vi "RS485_Sensor_Data.vi"() -> ()   [LabVIEW 2016]
uses:
  <vilib>/Instr/_visa.llb/VISA Set IO Buffer Mask.ctl
  <vilib>/Instr/_visa.llb/VISA Flush IO Buffer Mask.ctl
  <vilib>/Analysis/NI_AALBase.lvlib
  GEN_2.lvlib
  <vilib>/Instr/_visa.llb/VISA Configure Serial Port (Instr).vi
  <vilib>/Analysis/1siggen.llb/Ramp Pattern by Delta.vi
  Sensor_GEN2_Config_Addr.ctl
  Sensor_GEN2_Stat_Addr.ctl
panel:
  in  "Limits 2":cluster{"F0":sgl, "F1":sgl}={"F0"=-0.5925, "F1"=-0.5925}
  in  "Write_Scales":bool
  in  "Write_offsets":bool
  in  "Limits":cluster{"F0":sgl, "F1":sgl}={"F0"=-62.0, "F1"=-401.0}
  in  "Write Configs":bool
  out "Theta_dot":cluster{"Mean":dbl, "Std":dbl}={"Mean"=nan, "Std"=-0.0} {"Std" format="%.4f"; "Mean" format="%.4f"}
  out "Sum":cluster{"Mean":dbl, "Std":dbl}={"Mean"=-0.5323241930454969, "Std"=0.5862224441831317} {"Std" format="%.4f"; "Mean" format="%.4f"}
  out "F1":cluster{"Mean":dbl, "Std":dbl}={"Mean"=0.0509179662913084, "Std"=0.4077269270042539} {"Std" format="%.4f"; "Mean" format="%.4f"}
  in  "MT":cluster{"Expected":sgl, "Tolerance":sgl}
  in  "Find MT":bool
  out "Errors":bool[](array[boolean])
  in  "All config":cluster{"Config Address 2":T1, dbl}[](array[cluster])=[{"Config Address 2"=0, 66.0}, {"Config Address 2"=1, 0.0}, {"Config Address 2"=2, 8000000.0}, {"Config Address 2"=3, -62.0}, {"Config Address 2"=4, -0.5924999713897705}, {"Config Address 2"=5, -401.0}, {"Config Address 2"=6, -0.5924999713897705}, {"Config Address 2"=7, 0.0}, {"Config Address 2"=8, 0.0}, {"Config Address 2"=9, 0.0}, {"Config Address 2"=10, 0.0}, {"Config Address 2"=11, 0.0}, {"Config Address 2"=12, 0.0}, {"Config Address 2"=13, 0.0}, {"Config Address 2"=14, 0.0}, {"Config Address 2"=15, 0.0}, {"Config Address 2"=16, 0.0}, {"Config Address 2"=17, 0.0}, {"Config Address 2"=18, 0.0}, {"Config Address 2"=19, 0.0}, {"Config Address 2"=20, 0.0}, {"Config Address 2"=21, 0.0}, {"Config Address 2"=22, 0.0}, {"Config Address 2"=23, 0.0}, {"Config Address 2"=24, 0.0}, {"Config Address 2"=25, 0.0}, {"Config Address 2"=26, 0.0}, {"Config Address 2"=27, 0.0}, {"Config Address 2"=28, 0.0}] {"Config Address 2" items=["ID", "Mode", "Baudrate", "F0_Offset", "F0_Scale", "F1_Offset", "F1_Scale", "Iq P gain", "Iq I gain", "Iq D gain", "Velo P gain", "Velo I gain", "Velo D gain", "Posi P gain", "Posi I gain", "Posi D gain", "DirectForce P", "DirectForce I", "DirectForce D", "Limit Id Max", "Limit Iq Max", "Limit Velo Max", "Limit Posi Min", "Limit Posi Max", "Voltage Min", "Voltage Max", "Watchdog", "Temperature Low", "Temperature High"]}
  in  "SAVE":bool
  out "Vbus":dbl(graph)=11.947348594665527
  out "Error count":u64=15808
  in  "Read Configs":bool
  out "Temperature":cluster{dbl, dbl, dbl}(graph)={32.0, 38.6953125, 40.8125}
  out "Iq":cluster{dbl, dbl}(graph)={-0.5924999713897705, -0.5924999713897705}
  out "F0F1":cluster{dbl, dbl}(graph)={-0.5924999713897705, -0.0}
  out "Theta":cluster{dbl, dbl}(graph)={1.6263460338450386e-06, -5.619574039883446e-06}
  out "Theta_dot":cluster{dbl, dbl}(graph)={0.0024718716740608215, -0.0008698757737874985}
  in  "ID":u8=66
  in  "Read":bool=TRUE
  out "Theta_LP":sgl=1.626346e-06
  in  "Write_Mode":bool
  in  "Mode":i32(listbox)=2
  out "F0":cluster{"Mean":dbl, "Std":dbl}={"Mean"=-0.5832421593368053, "Std"=0.419881204420701} {"Std" format="%.4f"; "Mean" format="%.4f"}
  in  "stop":bool
  in  "Baudrate":u32=8000000
  in  "Buffer Size":u32=150000
  in  "COM":refnum<visa-resource-name>="COM10"
  # "0: WARN COMM\n1: WARN OVTEMP\n2: ERR ABS POSI\n3: ERR WTCHDOG\n4: ERR JOINT LMT\n5: ERR HW FAULT\n6: ERR INIT"
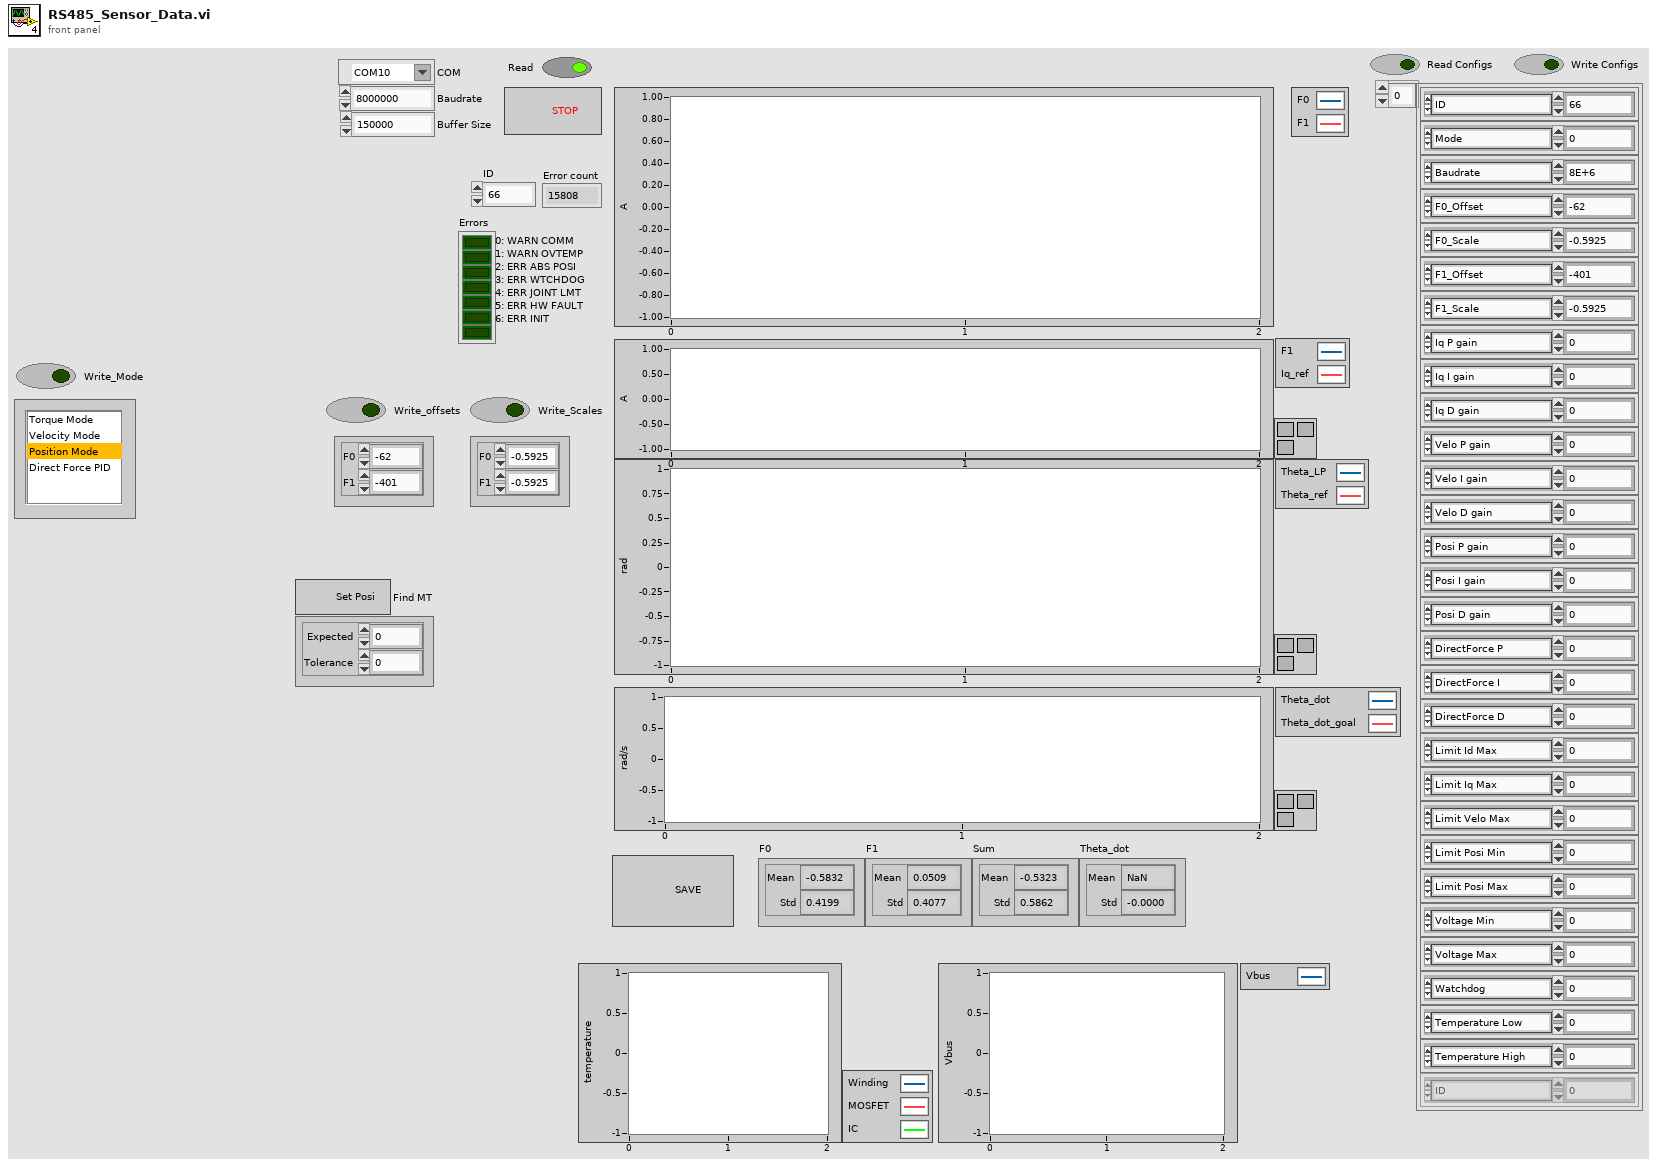
[diagram p1: front panel]
types:
  T1 = typedef "GEN_2.lvlib/Sensor_GEN2_Config_Addr.ctl" = u8
  T2 = typedef "VISA Flush IO Buffer Mask.ctl" = u16
  T3 = typedef "VISA Set IO Buffer Mask.ctl" = u16
  T4 = typedef "GEN_2.lvlib/Sensor_GEN2_Stat_Addr.ctl" = u8
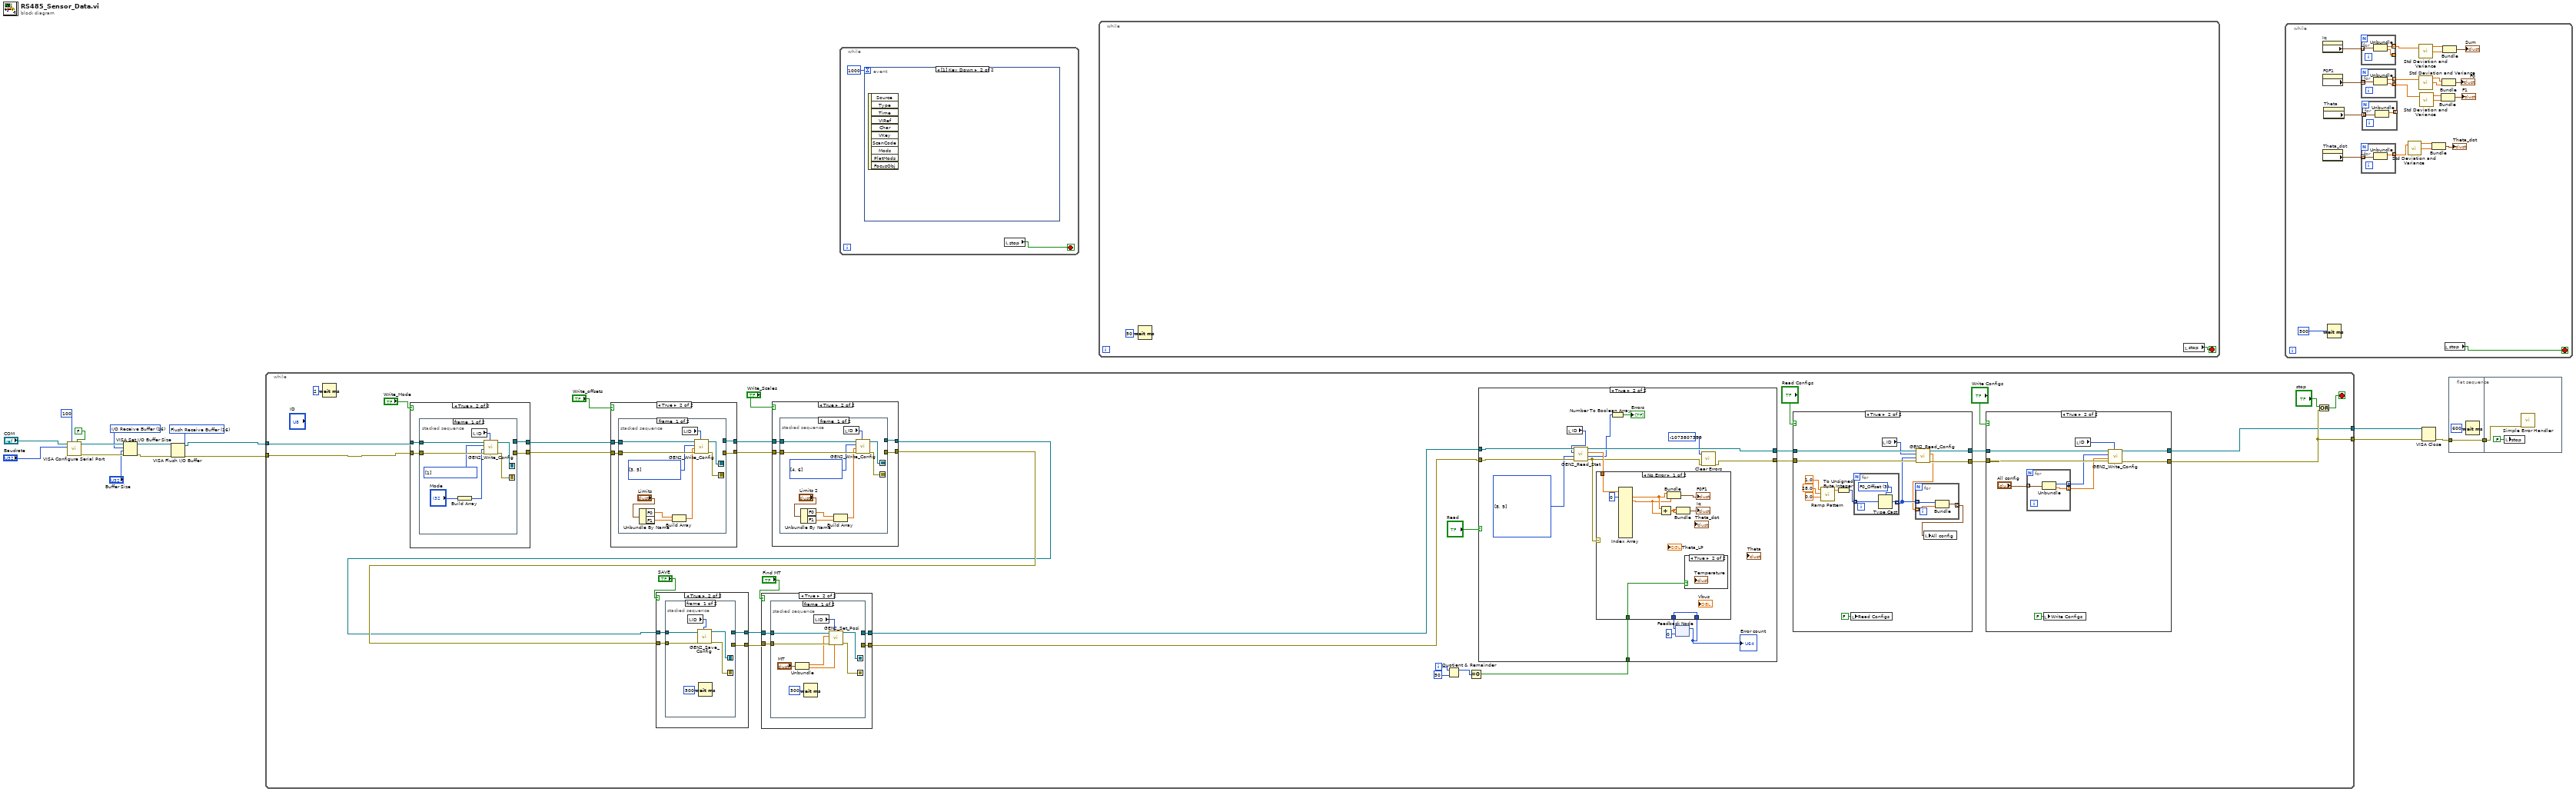
[diagram p0: block diagram]
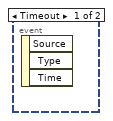
[diagram p2: hidden frame]
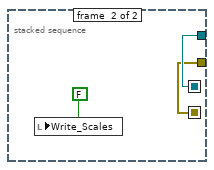
[diagram p4: hidden frame]
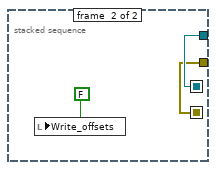
[diagram p6: hidden frame]
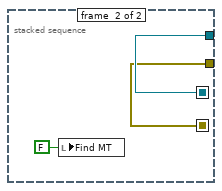
[diagram p9: hidden frame]
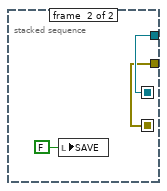
[diagram p11: hidden frame]
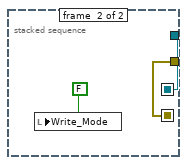
[diagram p14: hidden frame]
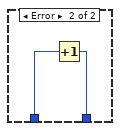
[diagram p17: hidden frame]
diagram:
  w3 = T2 16 items=["Flush Receive Buffer"=16, "Write Transmit Buffer to Device"=32, "Flush Receive Buffer (No I/O)"=64, "Flush Transmit Buffer"=128] ("Mask")
  w5 = T3 16 items=["I/O Receive Buffer"=16, "I/O Transmit Buffer"=32, "I/O Receive and Transmit Buffer"=48] ("Mask")
  n1 = call-poly "VISA Configure Serial Port"("VISA resource name"="COM", "timeout (10sec)"=u32 100, "Enable Termination\nChar (T)"=FALSE ("Enable Termination\nChar (T)"), "baud rate (9600)"="Baudrate") -> ("VISA resource name out"=w12:refnum<visa-resource-name>, "error out"=w11:errorcluster)  [unwired: 10 in]
  n2 = VISA Set I/O Buffer Size(VISA resource name=w12, mask (16)=w5, size (4096)="Buffer Size", error in (no error)=w11) -> (VISA resource name out=w1:refnum<visa-resource-name>, error out=w2:errorcluster)
  n3 = VISA Flush I/O Buffer(VISA resource name=w1, mask (16)=w3, error in (no error)=w2) -> (VISA resource name out=w6:refnum<visa-resource-name>, error out=w9:errorcluster)
  n4 = while {
    tunnel: w6 -> [w26]
    tunnel: w9 -> [w27]
    tunnel: [w31] -> w15
    tunnel: [w32] -> w14
    i -> [w36]
    stop <- w49 stop-if-true
    n5 = Wait (ms)(milliseconds to wait=u32 2) -> ()  [unwired: 1 out]
    n6 = case shown="True" "Write_Mode" {
      tunnel: w27 -> [w159 w163]
      tunnel: w26 -> [w158 w162]
      tunnel: [w159 w161] -> w23
      tunnel: [w158 w160] -> w24
      frame False {
      }
      frame True {
        n7 = stacked-sequence {
          seq-local: [w167 _] -> [_ w173]
          seq-local: [w168 _] -> [_ w172]
          tunnel: w163 -> [w169 _]
          tunnel: w162 -> [w170 _]
          tunnel: [_ w172] -> w161
          tunnel: [_ w173] -> w160
          frame #0 {
            w164 = T1[] [1] items=["ID", "Mode", "Baudrate", "F0_Offset", "F0_Scale", "F1_Offset", "F1_Scale", "Iq P gain", "Iq I gain", "Iq D gain", "Velo P gain", "Velo I gain", "Velo D gain", "Posi P gain", "Posi I gain", "Posi D gain", "DirectForce P", "DirectForce I", "DirectForce D", "Limit Id Max", "Limit Iq Max", "Limit Velo Max", "Limit Posi Min", "Limit Posi Max", "Voltage Min", "Voltage Max", "Watchdog", "Temperature Low", "Temperature High"] ("Config Addr")
            n8 = Build Array("Mode") -> (w166:i32[])
            n9 = local read "ID"() -> (w171:u8)
            n10 = call "GEN2_Write_Config.vi"("ID"=w171, "error in (no error)"=w169, "Data"=w166, "Config Addr"=w164, "VISA Refnum in"=w170) -> ("error out"=w168:errorcluster, "VISA Refnum out"=w167:refnum<visa-resource-name>)  [unwired: 5 in]
          }
          frame #1 {
            n11 = local write "Write_Mode"(FALSE ("WriteP_PID")) -> ()
          }
        }
      }
    }
    n12 = case shown="True" "Write_offsets" {
      tunnel: w23 -> [w71 w75]
      tunnel: w24 -> [w70 w74]
      tunnel: [w71 w73] -> w20
      tunnel: [w70 w72] -> w19
      frame False {
      }
      frame True {
        n13 = stacked-sequence {
          seq-local: [w82 _] -> [_ w87]
          seq-local: [w81 _] -> [_ w86]
          tunnel: w75 -> [w80 _]
          tunnel: w74 -> [w83 _]
          tunnel: [_ w86] -> w73
          tunnel: [_ w87] -> w72
          frame #0 {
            w76 = T1[] [3, 5] items=["ID", "Mode", "Baudrate", "F0_Offset", "F0_Scale", "F1_Offset", "F1_Scale", "Iq P gain", "Iq I gain", "Iq D gain", "Velo P gain", "Velo I gain", "Velo D gain", "Posi P gain", "Posi I gain", "Posi D gain", "DirectForce P", "DirectForce I", "DirectForce D", "Limit Id Max", "Limit Iq Max", "Limit Velo Max", "Limit Posi Min", "Limit Posi Max", "Voltage Min", "Voltage Max", "Watchdog", "Temperature Low", "Temperature High"] ("Config Addr")
            n14 = Unbundle By Name("Limits") -> ("F0"=w77:sgl, "F1"=w78:sgl)
            n15 = Build Array(w77, w78) -> (w79:sgl[])
            n16 = local read "ID"() -> (w84:u8)
            n17 = call "GEN2_Write_Config.vi"("ID"=w84, "error in (no error)"=w80, "Data"=w79, "Config Addr"=w76, "VISA Refnum in"=w83) -> ("error out"=w81:errorcluster, "VISA Refnum out"=w82:refnum<visa-resource-name>)  [unwired: 5 in]
          }
          frame #1 {
            n18 = local write "Write_offsets"(FALSE ("WriteP_PID")) -> ()
          }
        }
      }
    }
    n19 = case shown="True" "Write_Scales" {
      tunnel: w20 -> [w52 w56]
      tunnel: w19 -> [w51 w55]
      tunnel: [w52 w54] -> w21
      tunnel: [w51 w53] -> w18
      frame False {
      }
      frame True {
        n20 = stacked-sequence {
          seq-local: [w63 _] -> [_ w68]
          seq-local: [w62 _] -> [_ w67]
          tunnel: w56 -> [w61 _]
          tunnel: w55 -> [w64 _]
          tunnel: [_ w67] -> w54
          tunnel: [_ w68] -> w53
          frame #0 {
            w57 = T1[] [4, 6] items=["ID", "Mode", "Baudrate", "F0_Offset", "F0_Scale", "F1_Offset", "F1_Scale", "Iq P gain", "Iq I gain", "Iq D gain", "Velo P gain", "Velo I gain", "Velo D gain", "Posi P gain", "Posi I gain", "Posi D gain", "DirectForce P", "DirectForce I", "DirectForce D", "Limit Id Max", "Limit Iq Max", "Limit Velo Max", "Limit Posi Min", "Limit Posi Max", "Voltage Min", "Voltage Max", "Watchdog", "Temperature Low", "Temperature High"] ("Config Addr")
            n21 = Unbundle By Name("Limits 2") -> ("F0"=w58:sgl, "F1"=w59:sgl)
            n22 = Build Array(w58, w59) -> (w60:sgl[])
            n23 = local read "ID"() -> (w65:u8)
            n24 = call "GEN2_Write_Config.vi"("ID"=w65, "error in (no error)"=w61, "Data"=w60, "Config Addr"=w57, "VISA Refnum in"=w64) -> ("error out"=w62:errorcluster, "VISA Refnum out"=w63:refnum<visa-resource-name>)  [unwired: 5 in]
          }
          frame #1 {
            n25 = local write "Write_Scales"(FALSE ("WriteP_PID")) -> ()
          }
        }
      }
    }
    n26 = case shown="True" "SAVE" {
      tunnel: w18 -> [w122 w126]
      tunnel: w21 -> [w121 w124]
      tunnel: [w122 w125] -> w41
      tunnel: [w121 w123] -> w40
      frame False {
      }
      frame True {
        n27 = stacked-sequence {
          seq-local: [w130 _] -> [_ w135]
          seq-local: [w128 _] -> [_ w134]
          tunnel: w126 -> [w132 _]
          tunnel: w124 -> [w129 _]
          tunnel: [_ w135] -> w125
          tunnel: [_ w134] -> w123
          frame #0 {
            n28 = local read "ID"() -> (w131:u8)
            n29 = call "GEN2_Save_Config.vi"("ID"=w131, "error in (no error)"=w129, "VISA Refnum in"=w132) -> ("error out"=w128:errorcluster, "VISA Refnum out"=w130:refnum<visa-resource-name>)  [unwired: 7 in]
            n30 = Wait (ms)(milliseconds to wait=u32 500) -> ()  [unwired: 1 out]
          }
          frame #1 {
            n31 = local write "SAVE"(FALSE ("SAVE")) -> ()
          }
        }
      }
    }
    n32 = case shown="True" "Find MT" {
      tunnel: w41 -> [w104 w108]
      tunnel: w40 -> [w103 w105]
      tunnel: [w104 w107] -> w39
      tunnel: [w103 w106] -> w38
      frame False {
      }
      frame True {
        n33 = stacked-sequence {
          seq-local: [w116 _] -> [_ w120]
          seq-local: [w115 _] -> [_ w119]
          tunnel: w108 -> [w114 _]
          tunnel: [_ w120] -> w107
          tunnel: [_ w119] -> w106
          tunnel: w105 -> [w113 _]
          frame #0 {
            n34 = Unbundle("MT") -> ("Expected"=w111:sgl, "Tolerance"=w110:sgl)
            n35 = Wait (ms)(milliseconds to wait=u32 500) -> ()  [unwired: 1 out]
            n36 = local read "ID"() -> (w109:u8)
            n37 = call "GEN2_Set_Posi.vi"("Tolerance"=w110, "ID"=w109, "error in (no error)"=w113, "Expected Theta"=w111, "VISA Refnum in"=w114) -> ("error out"=w115:errorcluster, "VISA Refnum out"=w116:refnum<visa-resource-name>)  [unwired: 5 in]
          }
          frame #1 {
            n38 = local write "Find MT"(FALSE ("SAVE")) -> ()
          }
        }
      }
    }
    n39 = Quotient & Remainder(x=w36, y=50) -> (x-y*floor(x/y)=w34:i32)  [unwired: 1 out]
    n40 = Equal To 0?(x=w34) -> (x = 0?=w33:bool)
    n41 = case shown="True" "Read" {
      tunnel: [w176 w187] -> w43
      tunnel: w38 -> [w175 w190]
      tunnel: w39 -> [w176 w191]
      tunnel: [w175 w184] -> w44
      tunnel: w33 -> [_ w178]
      frame False {
      }
      frame True {
        w177 = T4[] [8, 9] items=["Torque Enable", "Homing Complete", "F0", "F1", "Goal Velo", "Goal Posi", "Present Id", "Present Iq", "Present Velo", "Present Posi", "Bus Voltage", "Temperature Winding", "Temperature MOSFET", "Temperature IC", "Error Status", "Iq_Temps"]
        n42 = local read "ID"() -> (w189:u8)
        n43 = call "GEN2_Read_Stat.vi"("error in (no error)"=w190, "Stat Address"=w177, "ID"=w189, "VISA Refnum in"=w191) -> ("error out"=w185:errorcluster, "ERROR"=w180:u8, "Data"=w188:dbl[], "VISA Refnum out"=w187:refnum<visa-resource-name>)  [unwired: 4 in]
        n44 = Number To Boolean Array(number=w180) -> (Boolean array=→"Errors":bool[])
        n45 = feedback #1(u64 0) -> (w182:u64)
        n46 = case shown="No Error" w185 {
          tunnel: w188 -> [w198 _]
          tunnel: w182 -> [w197 w202]
          tunnel: [w197 w201] -> w181
          tunnel: w178 -> [w196 _]
          frame No Error {
            n47 = Index Array(array=w198, index #1=0 ("index")) -> (element #1=w195:dbl, element #2=w194:dbl)  [unwired: 11 in, 10 out]
            n48 = Add(x=w195, y=w194) -> (x+y=w193:dbl)
            n49 = Bundle(w195, w194) -> (→"F0F1":cluster{dbl, dbl})  [unwired: 1 in]
            n50 = Bundle(w193, w193) -> (→"Iq":cluster{dbl, dbl})  [unwired: 1 in]
            n51 = case shown="True" w196 {
              frame False {
              }
              frame True {
              }
            }
          }
          frame Error {
            n52 = Increment(x=w202) -> (x+1=w201:u64)
          }
        }
        "Error count" <- w181
        n53 = feedback-in #1(w181) -> ()
        n54 = call <vilib>:"Clear Errors.vi"("error in (no error)"=w185, "specific error code to clear (0: all)"=-1073807339) -> ("error out"=w184:errorcluster)  [unwired: 4 in, 1 out]
      }
    }
    n55 = case shown="True" "Read Configs" {
      tunnel: w44 -> [w136 w150]
      tunnel: w43 -> [w137 w149]
      tunnel: [w136 w147] -> w29
      tunnel: [w137 w146] -> w30
      frame False {
      }
      frame True {
        n56 = call-poly <vilib>:"Ramp Pattern.vi"("start"=0.0, "end"=28.0, "delta"=1.0) -> ("Ramp Pattern"=w142:dbl[])  [unwired: 6 in, 2 out]
        n57 = To Unsigned Byte Integer(number=w142) -> (unsigned 8bit integer=w141:u8[])
        n58 = local write "Read Configs"(FALSE ("Read Config")) -> ()
        n59 = for {
          tunnel: w141 -> [w157] mode=indexing
          tunnel: [w156] -> w140 mode=indexing
          w155 = T1 3 items=["ID", "Mode", "Baudrate", "F0_Offset", "F0_Scale", "F1_Offset", "F1_Scale", "Iq P gain", "Iq I gain", "Iq D gain", "Velo P gain", "Velo I gain", "Velo D gain", "Posi P gain", "Posi I gain", "Posi D gain", "DirectForce P", "DirectForce I", "DirectForce D", "Limit Id Max", "Limit Iq Max", "Limit Velo Max", "Limit Posi Min", "Limit Posi Max", "Voltage Min", "Voltage Max", "Watchdog", "Temperature Low", "Temperature High"] ("Config Address")
          n60 = Type Cast(type=w155, x=w157) -> (*(type *) &x=w156:T1)
        }
        n61 = local read "ID"() -> (w148:u8)
        n62 = call "GEN2_Read_Config.vi"("error in (no error)"=w150, "Config Address"=w140, "ID"=w148, "VISA Refnum in"=w149) -> ("error out"=w147:errorcluster, "Data"=w139:dbl[], "VISA Refnum out"=w146:refnum<visa-resource-name>)  [unwired: 4 in, 1 out]
        n63 = for {
          tunnel: w140 -> [w154] mode=indexing
          tunnel: w139 -> [w153] mode=indexing
          tunnel: [w152] -> w138 mode=indexing
          n64 = Bundle("Config Address"=w154, w153) -> (w152:cluster{"Config Address":T1, dbl})  [unwired: 1 in]
        }
        n65 = local write "All config"(w138) -> ()
      }
    }
    n66 = case shown="True" "Write Configs" {
      tunnel: w29 -> [w89 w97]
      tunnel: w30 -> [w90 w98]
      tunnel: [w89 w95] -> w32
      tunnel: [w90 w96] -> w31
      frame False {
      }
      frame True {
        n67 = for {
          tunnel: "All config" -> [w102] mode=indexing
          tunnel: [w101] -> w92 mode=indexing
          tunnel: [w100] -> w91 mode=indexing
          n68 = Unbundle(w102) -> ("Config Address 2"=w101:T1, w100:dbl)
        }
        n69 = local write "Write Configs"(FALSE ("Read Config")) -> ()
        n70 = local read "ID"() -> (w94:u8)
        n71 = call "GEN2_Write_Config.vi"("ID"=w94, "error in (no error)"=w97, "Data"=w91, "Config Addr"=w92, "VISA Refnum in"=w98) -> ("error out"=w95:errorcluster, "VISA Refnum out"=w96:refnum<visa-resource-name>)  [unwired: 5 in]
      }
    }
    n72 = Or(x="stop", y=w32) -> (x .or. y?=w49:bool)
  }
  n73 = while {
    stop <- w204 stop-if-true
    n74 = event shown="[1] Key Down" {
      selector: _ -> [_ _]
      dyn-events: _ -> [_ _]
      timeout: 1000 -> [_ _]
      event Timeout {
        n75 = event-data() -> ()  [unwired: 1 in, 3 out]
      }
      event Key Down {
        n76 = event-data() -> ()  [unwired: 1 in, 10 out]
      }
    }
    n77 = local read "stop"() -> (w204:bool)
  }
  n78 = while {
    stop <- w206 stop-if-true
    n79 = Wait (ms)(milliseconds to wait=u32 50) -> ()  [unwired: 1 out]
    n80 = local read "stop"() -> (w206:bool)
  }
  n81 = while {
    stop <- w219 stop-if-true
    n82 = property on="Iq" class="WFChart (strict)"() -> ("History Data"=w228:cluster{dbl, dbl}[])  [unwired: 2 in, 2 out]
    n83 = property on="F0F1" class="WFChart (strict)"() -> ("History Data"=w227:cluster{dbl, dbl}[])  [unwired: 2 in, 2 out]
    n84 = property on="Theta_dot" class="WFChart (strict)"() -> ("History Data"=w216:cluster{dbl, dbl}[])  [unwired: 2 in, 2 out]
    n85 = property on="Theta" class="WFChart (strict)"() -> ("History Data"=w217:cluster{dbl, dbl}[])  [unwired: 2 in, 2 out]
    n86 = Wait (ms)(milliseconds to wait=u32 500) -> ()  [unwired: 1 out]
    n87 = for {
      tunnel: w228 -> [w238] mode=indexing
      tunnel: [w237] -> w207 mode=indexing
      tunnel: [w236] -> _ mode=indexing
      n88 = Unbundle(w238) -> (w237:dbl, w236:dbl)
    }
    n89 = for {
      tunnel: w227 -> [w235] mode=indexing
      tunnel: [w234] -> w209 mode=indexing
      tunnel: [w233] -> w208 mode=indexing
      n90 = Unbundle(w235) -> (w234:dbl, w233:dbl)
    }
    n91 = for {
      tunnel: w216 -> [w229] mode=indexing
      tunnel: [w230] -> w213 mode=indexing
      n92 = Unbundle(w229) -> (w230:dbl)  [unwired: 1 out]
    }
    n93 = for {
      tunnel: w217 -> [w231] mode=indexing
      tunnel: [w232] -> _ mode=indexing
      n94 = Unbundle(w231) -> (w232:dbl)  [unwired: 1 out]
    }
    n95 = call <vilib>:"Std Deviation and Variance.vi"("X"=w213) -> ("mean"=w215:dbl, "standard deviation"=w214:dbl)  [unwired: 1 in, 1 out]
    n96 = call <vilib>:"Std Deviation and Variance.vi"("X"=w207) -> ("mean"=w223:dbl, "standard deviation"=w224:dbl)  [unwired: 1 in, 1 out]
    n97 = call <vilib>:"Std Deviation and Variance.vi"("X"=w209) -> ("mean"=w226:dbl, "standard deviation"=w225:dbl)  [unwired: 1 in, 1 out]
    n98 = call <vilib>:"Std Deviation and Variance.vi"("X"=w208) -> ("mean"=w222:dbl, "standard deviation"=w221:dbl)  [unwired: 1 in, 1 out]
    n99 = Bundle("mean"=w215, "standard deviation"=w214) -> (→"Theta_dot":cluster{"mean":dbl, "standard deviation":dbl})  [unwired: 1 in]
    n100 = Bundle("mean"=w222, "standard deviation"=w221) -> (→"F1":cluster{"mean":dbl, "standard deviation":dbl})  [unwired: 1 in]
    n101 = Bundle("mean"=w226, "standard deviation"=w225) -> (→"F0":cluster{"mean":dbl, "standard deviation":dbl})  [unwired: 1 in]
    n102 = Bundle("mean"=w223, "standard deviation"=w224) -> (→"Sum":cluster{"mean":dbl, "standard deviation":dbl})  [unwired: 1 in]
    n103 = local read "stop"() -> (w219:bool)
  }
  n104 = VISA Close(VISA resource name=w15, error in (no error)=w14) -> (error out=w8:errorcluster)
  n105 = flat-sequence {
    tunnel: w8 -> [w240]
    tunnel: [w240] -> w7
    tunnel: w7 -> [w241]
    frame #0 {
      n106 = Wait (ms)(milliseconds to wait=u32 600) -> ()  [unwired: 1 out]
    }
    frame #1 {
      n107 = local write "stop"(FALSE ("stop")) -> ()
      n108 = call <vilib>:"Simple Error Handler.vi"("error in (no error)"=w241) -> ()  [unwired: 4 in, 5 out]
    }
  }
